vi "Store Static VI References for Subpanel.vi"(8 "error in (no error)":errorcluster, 11 "UserPwd DB Configuration in":refnum<class "UserPwd DB Configuration.lvclass">) -> (0 "error out":errorcluster, 3 "UserPwd DB Configuration out":refnum<class "UserPwd DB Configuration.lvclass">)   [LabVIEW 2016, in "UserPwd DB.lvlib" / "UserPwd DB Configuration.lvclass"]
uses:
  <userlib>/Common Components/UserPwd DB/UserPwd DB Config/UserPwd DB Configuration.lvclass
  <userlib>/Configuration Dialog Actor/Configuration.lvclass
  C:/Program Files (x86)/National Instruments/LabVIEW 2016/user.lib/Configuration Dialog Actor/Configuration.lvclass
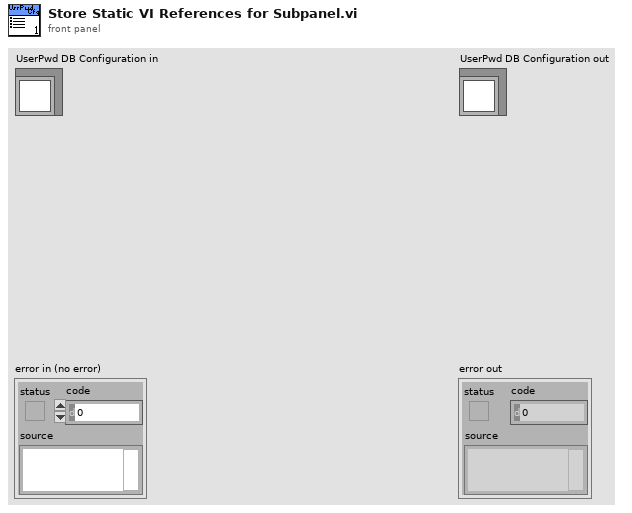
[diagram p1: front panel]
types:
  T1 = typedef "Configuration.lvlib/Configuration.lvclass/Data Retrieved by Lookup Table.ctl" = cluster{"VI Refnum":refnum<vi>, "Help Text":string}
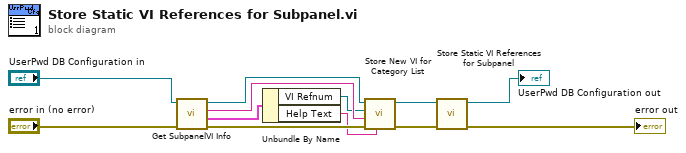
[diagram p0: block diagram]
diagram:
  n1 = call-dynamic "Get SubpanelVI Info.vi"("error in (no error)"="error in (no error)", "Configuration in"="UserPwd DB Configuration in") -> ("error out"=w9:errorcluster, "Subpanel VI data"=w3:T1, "Category string"=w4:string, "Configuration out"=w6:refnum<class "UserPwd DB Configuration.lvclass">)  [unwired: 6 in]
  n2 = Unbundle By Name(w3) -> ("VI Refnum"=w2:refnum<vi>, "Help Text"=w1:string)
  n3 = call <userlib>:"Store New VI for Category List.vi"("Help Text"=w1, "error in (no error)"=w9, "String"=w4, "VI Refnum"=w2, "Configuration in"=w6) -> ("error out"=w7:errorcluster, "Configuration out"=w5:refnum<class "UserPwd DB Configuration.lvclass">)  [unwired: 5 in]
  n4 = call-parent "Store Static VI References for Subpanel.vi"("error in (no error)"=w7, "Configuration in"=w5) -> ("error out"=→"error out":errorcluster, "Configuration out"=→"UserPwd DB Configuration out":refnum<class "UserPwd DB Configuration.lvclass">)  [unwired: 8 in]
